vi "Close.vi"(8 "error in (no error)":errorcluster, 11 "Oscilloscope in":refnum<class "Oscilloscope.lvclass">) -> (0 "error out":errorcluster, 3 "Oscilloscope out":refnum<class "Oscilloscope.lvclass">)   [LabVIEW 2020, in "Oscilloscope.lvclass"]
uses:
  Oscilloscope.lvclass
  C:/Code Projects/CircuitExplorer/AnalogDiscoveryFunction/AnalogDiscoveryFunction.lvclass
  AnalogDiscoveryFunction/AnalogDiscoveryFunction.lvclass/AnalogDiscoveryFunction.ctl
  AnalogDiscoveryFunction/GetInstrumentHandle.vi
  <vilib>/DigilentWF/DigilentWF.lvlib
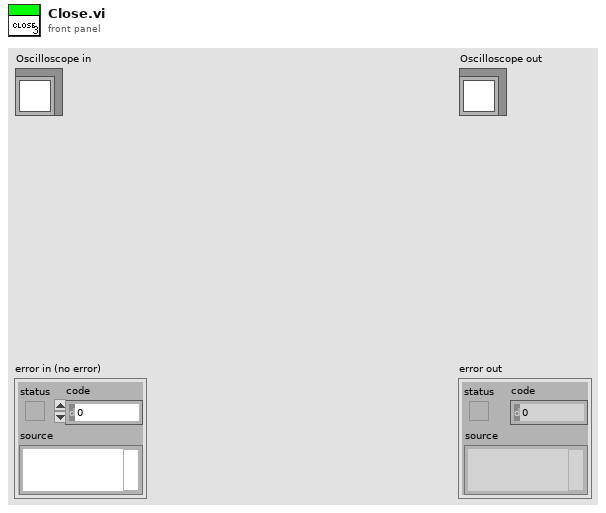
[diagram p1: front panel]
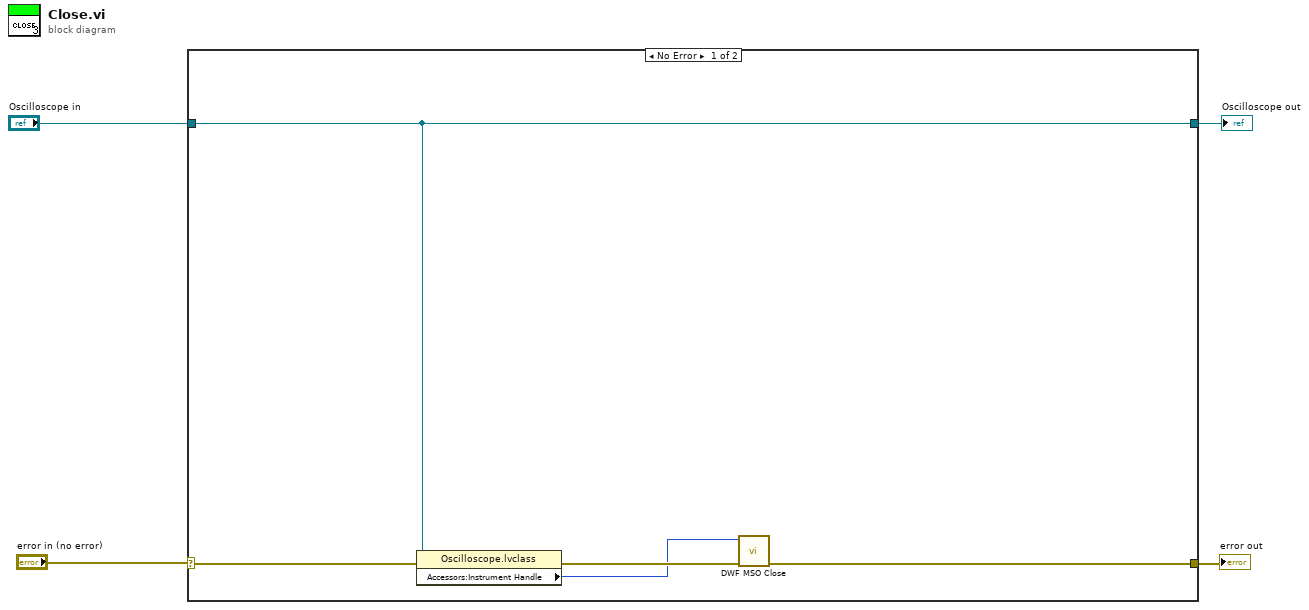
[diagram p0: block diagram]
diagram:
  n1 = case shown="No Error" "error in (no error)" {
    selector: "error in (no error)" -> [w9 w10]
    tunnel: [w6 w10] -> w1
    tunnel: [w5 w11] -> w2
    tunnel: "Oscilloscope in" -> [w5 w11]
    frame No Error {
      n2 = property class="Oscilloscope.lvclass"(reference=w5, error in=w9) -> (error out=w8:errorcluster, "Accessors:Instrument Handle"=w7:u32)  [unwired: 1 out]
      n3 = call <vilib>:"DWF MSO Close.vi"("Instrument Handle In"=w7, "Error In"=w8) -> ("Error Out"=w6:errorcluster)  [unwired: 13 in]
    }
    frame Error {
    }
  }
  "error out" <- w1
  "Oscilloscope out" <- w2
